vi "FunctionGenerator_Clear.vi"(11 "in FUNCTION_GENERATOR":T1) -> (3 "out FUNCTION_GENERATOR":T1)   [LabVIEW 2019, in "Trajectory_Library.lvlib"]
doc: "Clear out all entries.\n\nInputs:\n - \n\nOutputs:\n - Function Generator -- Created data structure"
uses:
  Trajectory_Library.lvlib
  FUNCTION_GENERATOR.ctl
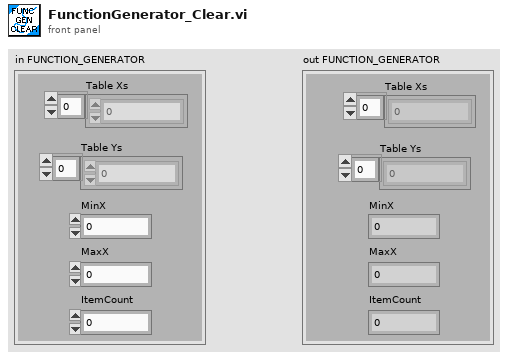
[diagram p1: front panel]
types:
  T1 = typedef "Trajectory_Library.lvlib/FUNCTION_GENERATOR.ctl" = cluster{"Table Xs":dbl[], "Table Ys":dbl[], "MinX":dbl, "MaxX":dbl, "ItemCount":i32}
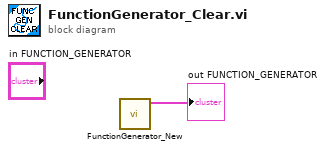
[diagram p0: block diagram]
diagram:
  n1 = call "FunctionGenerator_New.vi"() -> ("FUNCTION_GENERATOR"=→"out FUNCTION_GENERATOR":T1)  [unwired: 11 in]
